vi "Create Python Graph.vi"(0 "File Name":string, 1 "Init (F)":bool, 5 "Wet Test":bool, 7 "Y-Axis Max":i32, 11 "Error IN":errorcluster, 12 "Data Base Path":path, 13 "Python Script Directory":path=path "C:/Users/gtetil/Documents/Projects/ls-tester-graph-script", 14 "Data Start Index":u32) -> (4 "Command Line Error":string, 15 "Error OUT":errorcluster)   [LabVIEW 2013]
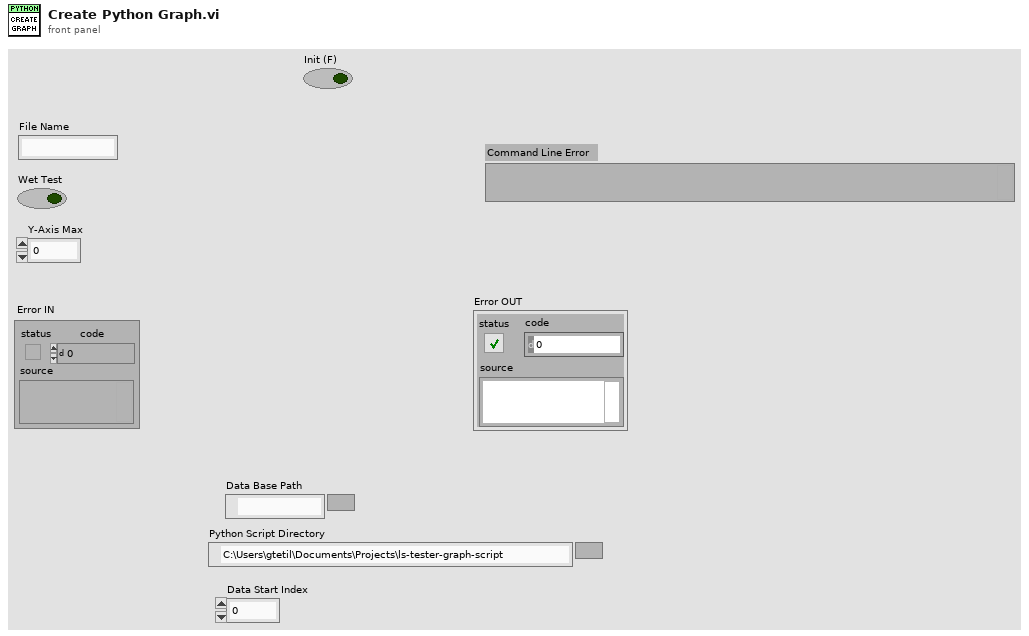
[diagram p1: front panel]
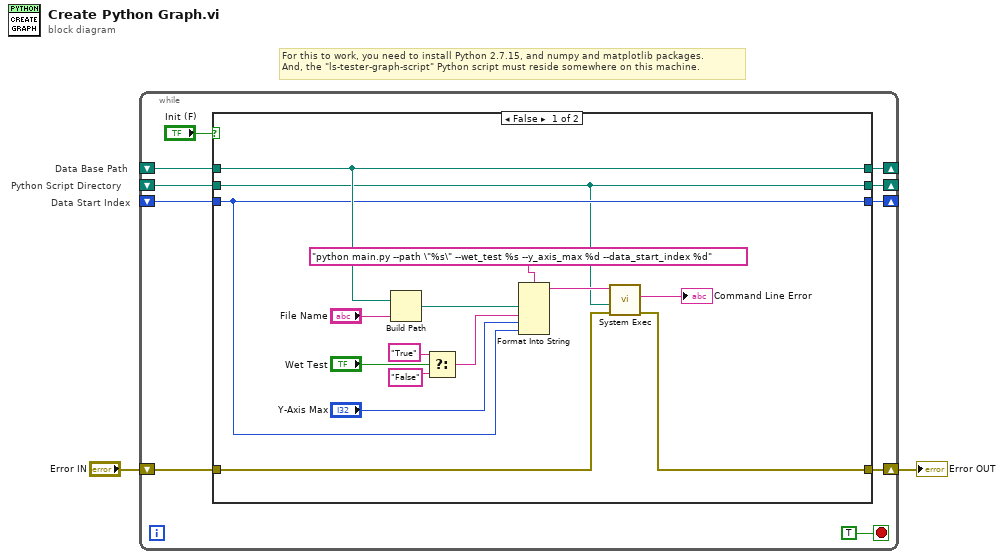
[diagram p0: block diagram]
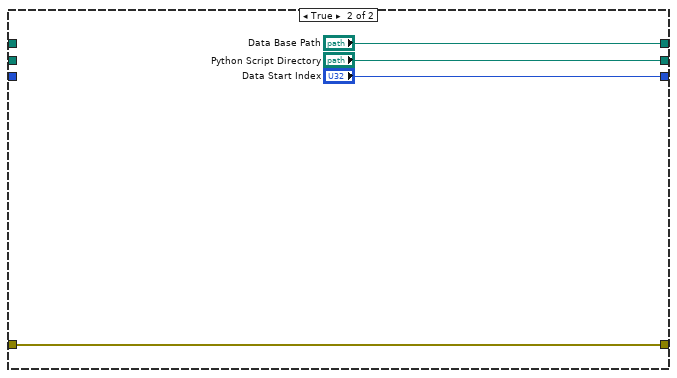
[diagram p2: hidden frame]
diagram:
  # "For this to work, you need to install Python 2.7.15, and numpy and matplotlib packages.\nAnd, the \"ls-tester-graph-script\" Python script must reside somewhere on this machine."
  # "Data Start Index"
  # "Python Script Directory"
  # "Data Base Path"
  n1 = while {
    shift-right: [w10] -> _
    shift-left: _ -> [w7]
    shift-right: [w9] -> _
    shift-left: _ -> [w6]
    shift-right: [w8] -> _
    shift-left: _ -> [w5]
    shift-right: [w3] -> w1
    shift-left: "Error IN" -> [w4]
    stop <- TRUE stop-if-true
    n2 = case shown="False" "Init (F)" {
      tunnel: [w18 "Data Base Path"] -> w10
      tunnel: [w16 "Python Script Directory"] -> w9
      tunnel: [w17 "Data Start Index"] -> w8
      tunnel: w7 -> [w18 _]
      tunnel: w6 -> [w16 _]
      tunnel: w5 -> [w17 _]
      tunnel: w4 -> [w15 w28]
      tunnel: [w14 w28] -> w3
      frame False {
        n3 = Build Path(base path=w18, name or relative path="File Name") -> (appended path=w20:path)
        n4 = Select(t="True", s="Wet Test", f="False") -> (s? t:f=w22:string)
        n5 = Format Into String(format string="python main.py --path \"%s\" --wet_test %s --y_axis_max %d --data_start_index %d", w20, w22, "Y-Axis Max", w17) -> (resulting string=w26:string)  [unwired: 2 in, 1 out]
        n6 = call <vilib>:"System Exec.vi"("error in (no error)"=w15, "working directory"=w16, "command line"=w26) -> ("error out"=w14:errorcluster, "standard error"=→"Command Line Error":string)  [unwired: 5 in, 2 out]
      }
      frame True {
      }
    }
  }
  "Error OUT" <- w1
